vi "DiscArchiver.register to event builder.vi"(0 "i ref in":refnum<vi>, 1 "collector":string, 2 "filePrefix":string, 3 "ms timeout (10000)":i32=10000, 4 "complete":bool, 5 "error in (no error)":errorcluster) -> (14 "i ref out":refnum<vi>, 17 "timed out":bool, 19 "error out":errorcluster)   [LabVIEW 2014, in "DiscArchiver.lvlib"]
doc: "Registers the archiver to an EventBuilder object and set the file body name."
uses:
  DiscArchiver.lvlib
  CS_Core/CAEObj/CAEObj.event definition.ctl
  CS_Core/CSSystem/CoreDefs/CoreDefs.error_type.ctl
  CS_Core/CAEObj/CAEObj.lvlib
  CS_Core/CSSystem/CoreLib/CoreLib.lvlib
panel:
  in  "event definition":T1
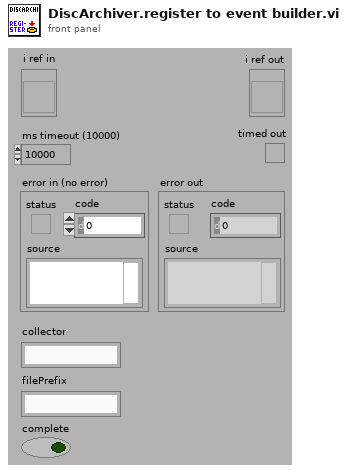
[diagram p1: front panel]
types:
  T1 = typedef "CAEObj.lvlib/CAEObj.event definition.ctl" = cluster{"URL":string, "enable":bool, "ignoreResID":bool}
  T2 = typedef "CoreDefs.error_type.ctl" = enum16{"no error", "can't load process", "can't unload process", "process does not exist", "can't install process", "can't remove process", "unknown function", "time out", "can't execute function", "duplicate queue name", "super not found", "caller queue invalid", "can't ping process", "unknown error", "VISA Error", "VISA timeout", "GPIB timeout", "GPIB error", "communication error", "data type mismatch", "can't read data from OPC server", "can't write data to OPC server", "OET error", "function not implemented", "process already exists", "invalid Shared Variable name", "error writing Shared Variable", "error reading Shared Variable", "invalid client name", "corrupt database", "unknown class", "call not authorized", "parameter out of range", "OET timeout: can't get data to modify", "invalid queue name", "requested operation incompatible with current state", "event undefined", "event disabled", "state undefined", "caller is not a friend", "EventBuilder: bad eventID", "EventBuilder: no DAQ devices", "a thread must not stop itself", "UNUSED ELEMENT4", "DiscArchiver: eventData incomplete", "DiscArchiver: eventData does not belong to run", "DiscArchiver: can't open file", "DiscArchiver: can't write to file", "DiscArchiver: available disc space low", "can't acquire semaphore", "error reading data from database", "notifier object is not existing", "can't register process", "can't unregister process", "illegal event type", "object disabled", "object already exists", "can't change state", "Instrument not found", "no connection to remote node", "invalid reference", "N/A", "UNUSED ELEMENT 1", "element not found", "illegal TCP/IP connection detected", "object does not exist", "invalid access ID", "unknown CS system", "invalid privilige", "unsupported data type", "unsupported server type", "IO server already exists", "Shared Variable already exists"}
  T3 = typedef "DiscArchiver.lvlib/DiscArchiver.i attribute.ctl" = cluster{"file prefix":string, "actual file":string, "nOfEvents":i32, "file":refnum<file>, "eventBuilder":string, "disc size alarm":bool, "dataDescription":string, "dataDescriptionURL":string, "eventDataURL":string, "headerID":dbl, "completeData":bool, "nOfEventsID":i32, "dataFileID":i32}
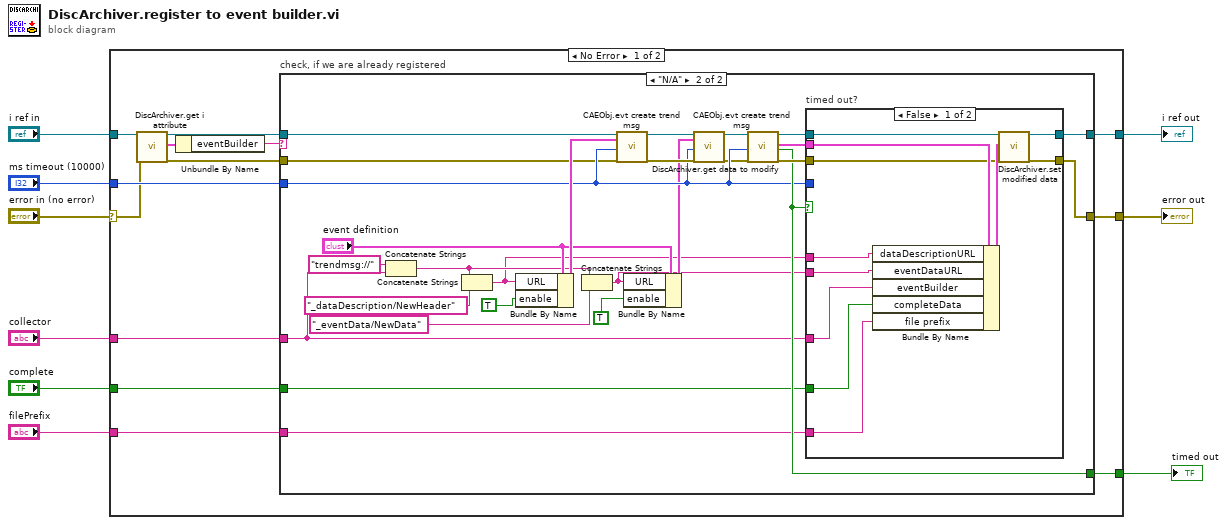
[diagram p0: block diagram]
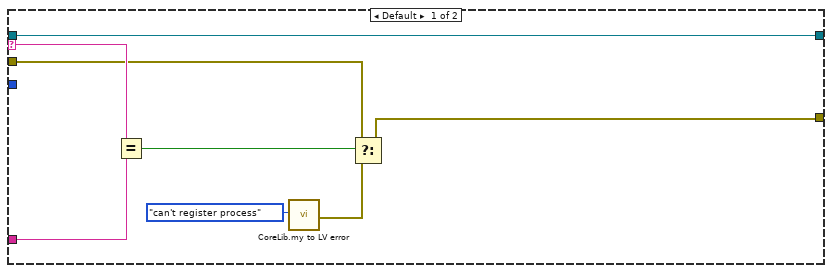
[diagram p2: hidden frame]
diagram:
  n1 = case shown="No Error" "error in (no error)" {
    selector: "error in (no error)" -> [w14 w71]
    tunnel: "i ref in" -> [w15 w72]
    tunnel: [w22 w72] -> w8
    tunnel: [w21 _] -> w7
    tunnel: "complete" -> [w20 _]
    tunnel: "collector" -> [w18 _]
    tunnel: "filePrefix" -> [w19 _]
    tunnel: [w16 w71] -> w3
    tunnel: "ms timeout (10000)" -> [w17 _]
    frame No Error {
      n2 = call "DiscArchiver.get i attribute.vi"("i ref in"=w15, "error in (no error)"=w14) -> ("i ref out"=w12:refnum<vi>, "i attribute"=w11:T3, "error out"=w13:errorcluster)  [unwired: 15 in]
      n3 = Unbundle By Name(w11) -> ("eventBuilder"=w10:string)
      n4 = case "check, if we are already registered" shown="\"N/A\"" w10 {
        selector: w10 -> [w28 _]
        tunnel: [w30 w57] -> w22
        tunnel: [_ w53] -> w21
        tunnel: w20 -> [_ w52]
        tunnel: w19 -> [_ w51]
        tunnel: w18 -> [w27 w49]
        tunnel: w17 -> [_ w43]
        tunnel: [w23 w35] -> w16
        tunnel: w13 -> [w24 w34]
        tunnel: w12 -> [w30 w33]
        frame Default {
          n5 = Equal?(x=w28, y=w27) -> (x = y?=w26:bool)
          n6 = call "CoreLib.my to LV error.vi"("ErrorTypes"=CoreDefs.error_type."can't register process") -> ("myErrorCluster"=w25:errorcluster)  [unwired: 17 in, 1 out]
          n7 = Select(t=w24, s=w26, f=w25) -> (s? t:f=w23:errorcluster)
        }
        frame "N/A" {
          n8 = Concatenate Strings("trendmsg://" ("string"), w49) -> (w38:string)
          n9 = Concatenate Strings(w38, "_dataDescription/NewHeader" ("string")) -> (w32:string)
          n10 = Bundle By Name(cluster="event definition", "URL"=w32, "enable"=TRUE) -> (w46:T1)
          n11 = Concatenate Strings(w38, "_eventData/NewData" ("string")) -> (w31:string)
          n12 = call "CAEObj.evt create trend msg.vi"("i ref in"=w33, "event definition"=w46, "ms timeout (10000)"=w43, "error in (no error)"=w34) -> ("i ref out"=w45:refnum<vi>, "error out"=w44:errorcluster)  [unwired: 12 in, 2 out]
          n13 = Bundle By Name(cluster="event definition", "URL"=w31, "enable"=TRUE) -> (w39:T1)
          n14 = call "CAEObj.evt create trend msg.vi"("i ref in"=w45, "event definition"=w39, "ms timeout (10000)"=w43, "error in (no error)"=w44) -> ("i ref out"=w42:refnum<vi>, "error out"=w41:errorcluster)  [unwired: 12 in, 2 out]
          n15 = call "DiscArchiver.get data to modify.vi"("i ref in"=w42, "ms timeout (10000)"=w43, "error in (no error)"=w41) -> ("i ref out"=w56:refnum<vi>, "i attribute"=w54:T3, "timed out"=w53:bool, "error out"=w55:errorcluster)  [unwired: 13 in]
          n16 = case "timed out?" shown="False" w53 {
            tunnel: [w68 w69] -> w35
            tunnel: [w67 w70] -> w57
            tunnel: w56 -> [w64 w70]
            tunnel: w55 -> [w63 w69]
            tunnel: w54 -> [w66 _]
            tunnel: w52 -> [w59 _]
            tunnel: w49 -> [w58 _]
            tunnel: w51 -> [w62 _]
            tunnel: w43 -> [_ _]
            tunnel: w32 -> [w61 _]
            tunnel: w31 -> [w60 _]
            frame False {
              n17 = Bundle By Name(cluster=w66, "dataDescriptionURL"=w61, "eventDataURL"=w60, "eventBuilder"=w58, "completeData"=w59, "file prefix"=w62) -> (w65:T3)
              n18 = call "DiscArchiver.set modified data.vi"("i ref in"=w64, "i attribute"=w65, "error in (no error)"=w63) -> ("i ref out"=w67:refnum<vi>, "error out"=w68:errorcluster)  [unwired: 15 in]
            }
            frame True {
            }
          }
        }
      }
    }
    frame Error {
    }
  }
  "error out" <- w3
  "i ref out" <- w8
  "timed out" <- w7
